vi "STL quick viewer.vi"() -> ()   [LabVIEW 2017]
uses:
  <vilib>/Utility/miscctls.llb/LVRGBAColorTypeDef.ctl
  sub-VIs/Low level/Cross product 3D_3Dpf.vi
  sub-VIs/Low level/Unit vector_3Dpf.vi
  sub-VIs/Low level/Dot product_3Dpf.vi
panel:
  in  "Render mode":T1(ring)=enum."Polygons"
  out "N triangles":i32
  out "3D Picture":refnum<vi>(3d-picture)
  in  "STL geometry file path":path
  # "PN 21/11/17"
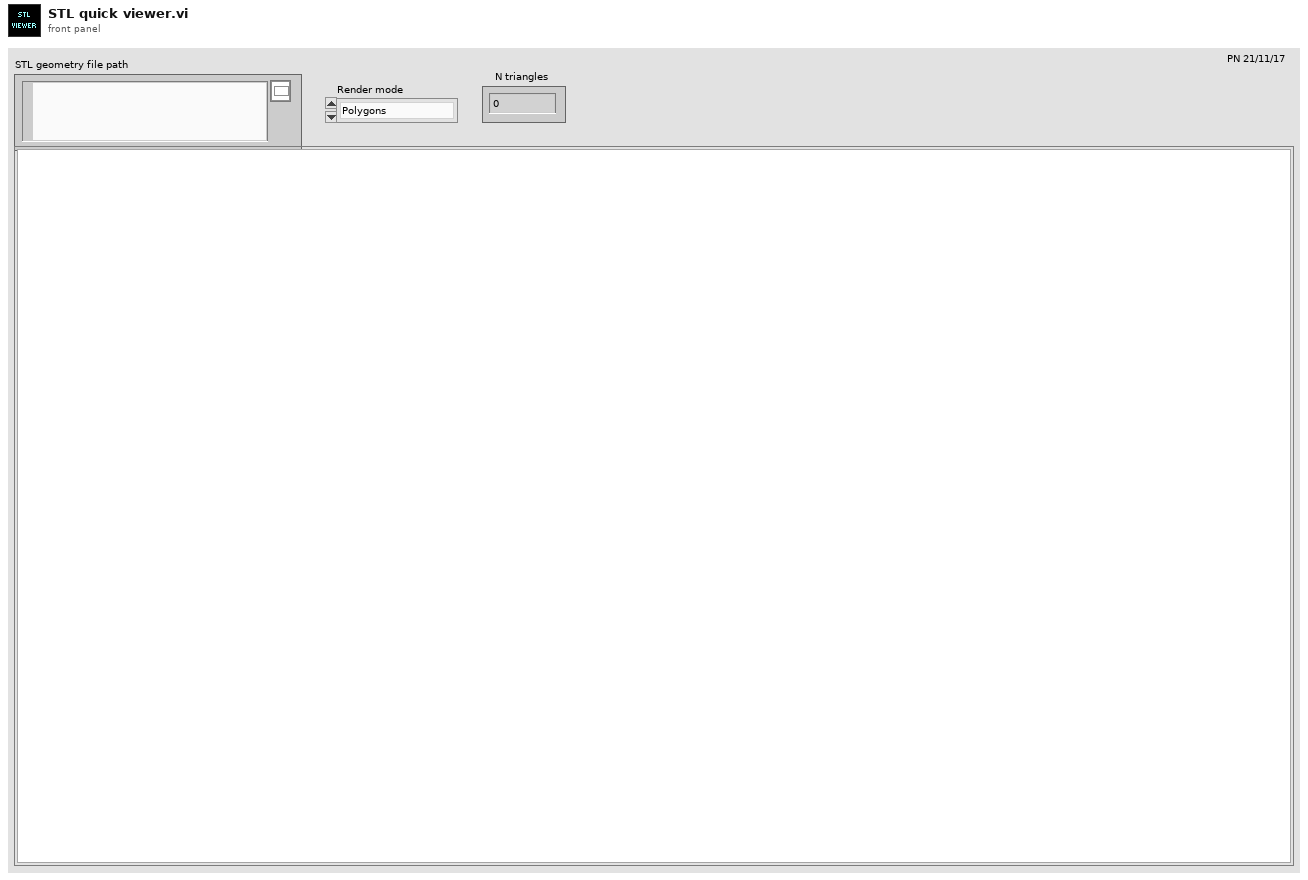
[diagram p1: front panel]
types:
  T1 = enum16{"Inherit Value", "Points", "Wireframe", "Polygons"}
  T2 = typedef "Triangle panel.ctl" = cluster{"V0":sgl[], "V1":sgl[], "V2":sgl[], "E0":sgl[], "E1":sgl[], "E2":sgl[], "n^":sgl[], "Pc":sgl[], "Gamma'":sgl, "V_transp.":sgl, "E0 link":i32, "E1 link":i32, "E2 link":i32}
  T3 = typedef "LVRGBAColorTypeDef.ctl" = cluster{"Red":sgl, "Green":sgl, "Blue":sgl, "Alpha":sgl}
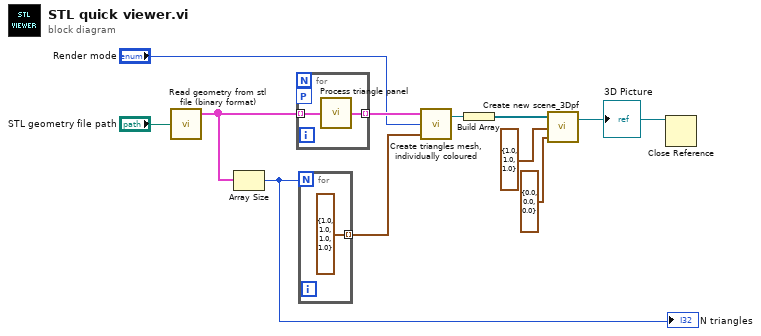
[diagram p0: block diagram]
diagram:
  n1 = call "Read geometry from stl file (binary format).vi"("STL file path"="STL geometry file path") -> ("Panel triangles array"=w3:T2[])  [unwired: 2 out]
  n2 = Array Size(array=w3) -> (size(s)=w2:i32)
  "N triangles" <- w2
  n3 = for {
    tunnel: w3 -> [w13] mode=indexing
    tunnel: [w12] -> w6 mode=indexing
    workers-P: _ -> [_]
    n4 = call "Process triangle panel.vi"("Panel triangle in"=w13) -> ("Panel triangle out"=w12:T2)
  }
  n5 = for {
    N: w2 -> [_]
    tunnel: [T3 {"Red"=1.0, "Green"=1.0, "Blue"=1.0, "Alpha"=1.0} ("Colour")] -> w4 mode=indexing
  }
  n6 = call "Create triangles mesh, individually coloured.vi"("Colours array"=w4, "Render mode"="Render mode", "Triangles array"=w6) -> ("Triangle mesh out"=w8:refnum<vi>)  [unwired: 1 out]
  n7 = Build Array(w8) -> (w7:refnum<vi>[])
  n8 = call "Create new scene_3Dpf.vi"("Translation"=cluster{"X":sgl, "Y":sgl, "Z":sgl} {"X"=0.0, "Y"=0.0, "Z"=0.0}, "Scale"=cluster{"X":sgl, "Y":sgl, "Z":sgl} {"X"=1.0, "Y"=1.0, "Z"=1.0}, "Scene objects array"=w7) -> ("Scene out"=w5:refnum<vi>)  [unwired: 1 out]
  "3D Picture" <- w5
  n9 = Close Reference(reference=w5) -> ()  [unwired: 1 in, 1 out]
